vi "unused_applyInsertSpace.vi"(4 "deltaY":u16, 6 "deltaX":u16, 8 "error in (no error)":errorcluster, 10 "origin":T1, 11 "AbstractDiagram in":refnum<class "AbstractDiagram.lvclass">) -> (0 "error out":errorcluster, 3 "AbstractDiagram out":refnum<class "AbstractDiagram.lvclass">)   [LabVIEW 2023]
uses:
  AbstractDiagram.lvclass/AbstractDiagram.ctl
  Ctrls/point.ctl
  TLC_Scripto.lvlib
  AbstractDiagram.lvclass
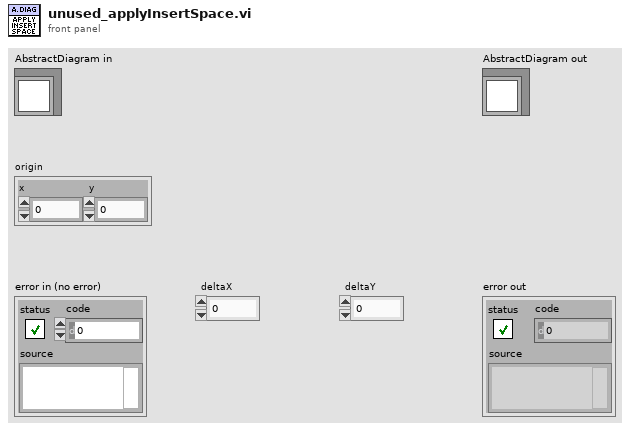
[diagram p1: front panel]
types:
  T1 = typedef "TLC_Scripto.lvlib/point.ctl" = cluster{"x":i32, "y":i32}
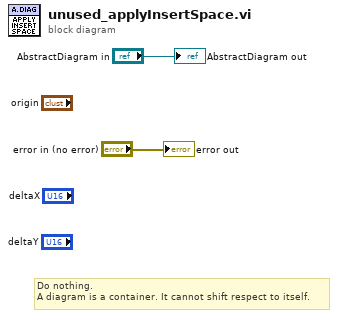
[diagram p0: block diagram]
diagram:
  # "Do nothing.\nA diagram is a container. It cannot shift respect to itself."
  "error out" <- "error in (no error)"
  "AbstractDiagram out" <- "AbstractDiagram in"
